vi "VESASignal_ScanNextVPixel.vi"(3 "Enable":bool) -> (15 "v_Pixel":i16)   [LabVIEW 2018]
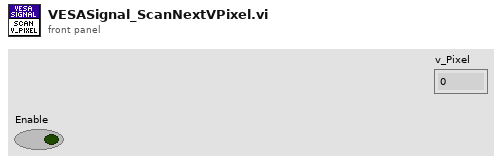
[diagram p1: front panel]
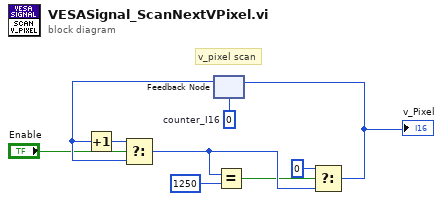
[diagram p0: block diagram]
diagram:
  w5 = i16 0  # counter_I16
  # "v_pixel scan"
  n1 = feedback #1(w5) -> (w9:i16)
  n2 = Increment(x=w9) -> (x+1=w7:i16)
  n3 = Select(t=w7, s="Enable", f=w9) -> (s? t:f=w8:i16)
  n4 = Equal?(x=w8, y=i16 1250) -> (x = y?=w6:bool)
  n5 = Select(t=i16 0 ("f"), s=w6, f=w8) -> (s? t:f=w1:i16)
  "v_Pixel" <- w1
  n6 = feedback-in #1(w1) -> ()
